vi "FT_Cycle_Port.vi"(1 "Handle":u32) -> (0 "FT_Status":u32)   [LabVIEW 2011]
uses:
  FTD2XX.dll
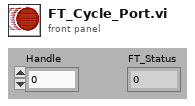
[diagram p1: front panel]
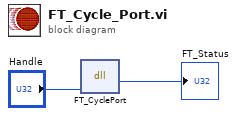
[diagram p0: block diagram]
diagram:
  n1 = dll-call lib="D:/WORK/LabView/#Avesta/D2XX_Functions_7.0/FTD2XX.dll" fn="FT_CyclePort"("Handle"="Handle") -> ("FT_Status"=→"FT_Status":u32)  [unwired: 4 in, 2 out]
